vi "find_rects_test.vi"() -> ()   [LabVIEW 2023]
uses:
  find_rects_parameters.ctl
  Vision.lvlib
panel:
  out "rects":T1(array[cluster]) {"x" format="%#_3g"; "y" format="%#_3g"; "width" format="%#_3g"; "height" format="%#_3g"; "angle" format="%#_3g"; "image-x" format="%#_3g"; "image-y" format="%#_3g"}
  in  "find_rects parameters":T2={"nominalWidth"=1.0, "nominalHeight"=1.0, "tolerance"=0.5, "pointSelect"=4.0, "allowRotation"=FALSE}
  in  "Field of View":cluster{"fieldOfViewX":sgl, "fieldOfViewY":sgl}={"fieldOfViewX"=1.4, "fieldOfViewY"=1.048}
  out "Number of Rects":i32
  in  "File Path":path=path "C:/Users/Caleb/Downloads/fid_range_test_br_7.png"
  out "error out":errorcluster
  out "Image":T3(plugin-control)
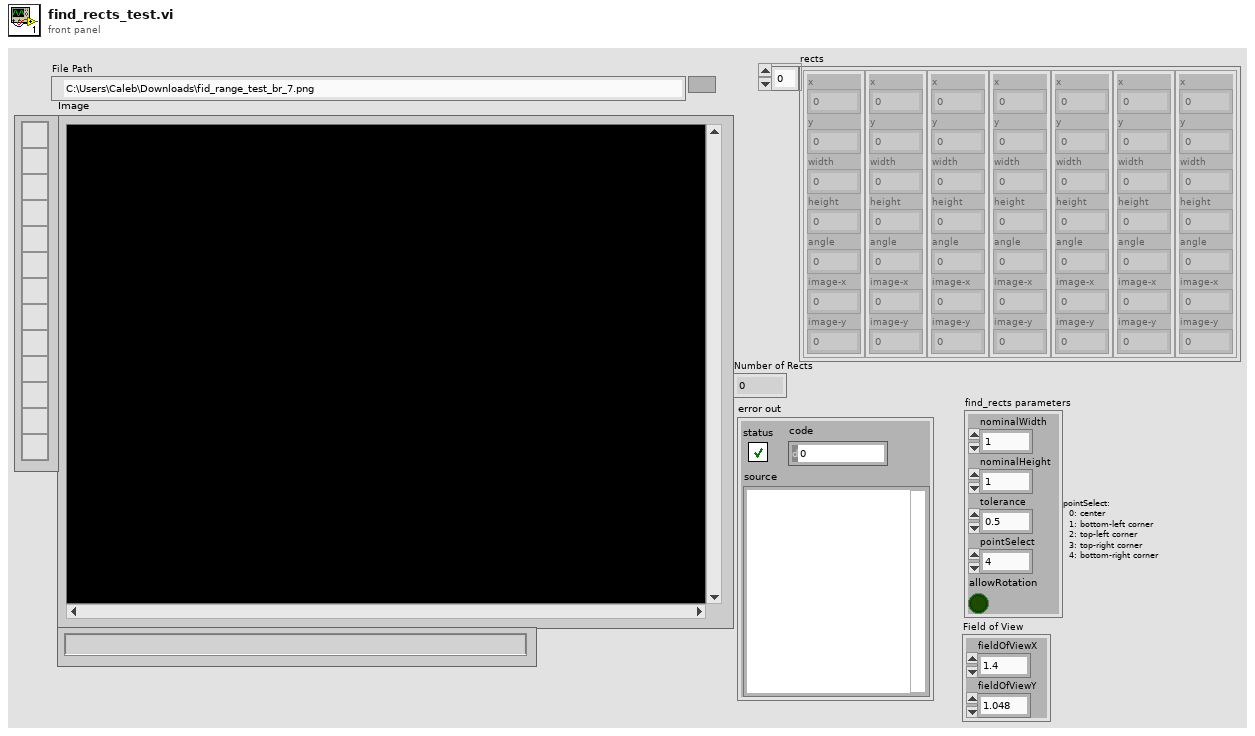
[diagram p1: front panel]
types:
  T1 = cluster{"x":dbl, "y":dbl, "width":dbl, "height":dbl, "angle":dbl, "image-x":dbl, "image-y":dbl}[]
  T2 = typedef "Vision.lvlib/find_rects_parameters.ctl" = cluster{"nominalWidth":sgl, "nominalHeight":sgl, "tolerance":sgl, "pointSelect":sgl, "allowRotation":bool}
  T3 = typedef "IMAQ Image.ctl" = refnum<image>
  T4 = cluster{"Left":i32, "Top":i32, "Right":i32, "Bottom":i32}
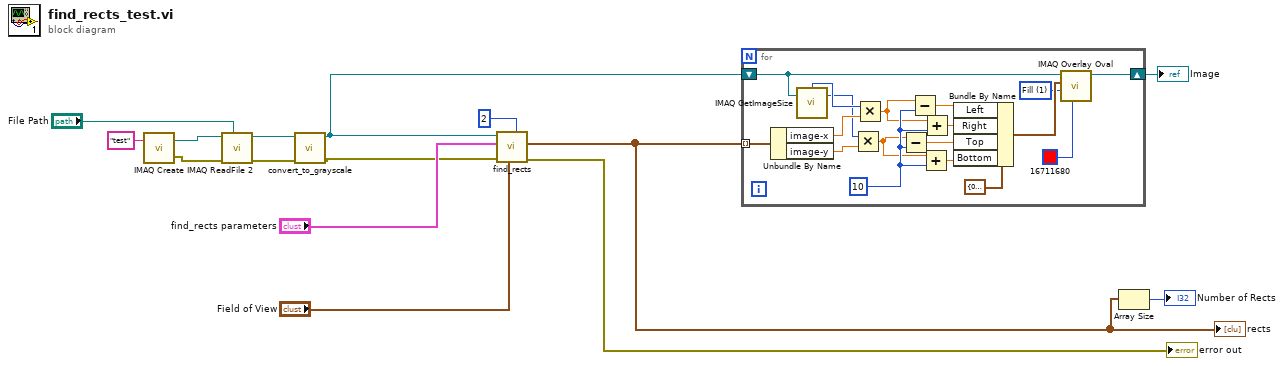
[diagram p0: block diagram]
diagram:
  n1 = call "IMAQ Create"("Image Name"="test") -> ("New Image"=w15:T3, "error out"=w13:errorcluster)  [unwired: 4 in]
  n2 = call "IMAQ ReadFile 2"("File Path"="File Path", "error in (no error)"=w13, "Image"=w15) -> ("error out"=w1:errorcluster, "Image Out"=w4:T3)  [unwired: 4 in, 3 out]
  n3 = call "convert_to_grayscale.vi"("error in (no error)"=w1, "Image in"=w4) -> ("error out"=w2:errorcluster, "Image out"=w3:T3)  [unwired: 8 in]
  n4 = call "find_rects.vi"("shrinkFactor"=2 ("Shrink Factor"), "Field of View"="Field of View", "error in"=w2, "find_patches parameters"="find_rects parameters", "Image"=w3) -> ("error out"=→"error out":errorcluster, "rects"=w5:T1)  [unwired: 5 in]
  "rects" <- w5
  n5 = for {
    shift-right: [w18] -> w7
    shift-left: w3 -> [w29]
    tunnel: w5 -> [w16] mode=indexing
    w17 = u32 1 items=["Frame", "Fill"] ("Drawing Mode (Frame)")
    w22 = 10
    n6 = Unbundle By Name(w16) -> ("image-x"=w33:dbl, "image-y"=w31:dbl)
    n7 = call "IMAQ GetImageSize"("Image"=w29) -> ("Y Resolution"=w30:i32, "X Resolution"=w32:i32)  [unwired: 3 in, 1 out]
    n8 = Multiply(x=w30, y=w31) -> (x*y=w21:dbl)
    n9 = Multiply(x=w32, y=w33) -> (x*y=w20:dbl)
    n10 = Subtract(x=w21, y=w22) -> (x-y=w23:dbl)
    n11 = Subtract(x=w20, y=w22) -> (x-y=w24:dbl)
    n12 = Add(x=w21, y=w22) -> (x+y=w25:dbl)
    n13 = Add(x=w20, y=w22) -> (x+y=w26:dbl)
    n14 = Bundle By Name(cluster=T4 {"Left"=0, "Top"=0, "Right"=0, "Bottom"=0} ("Bounding Rectangle"), "Left"=w24, "Right"=w26, "Top"=w23, "Bottom"=w25) -> (w19:T4)
    n15 = call "IMAQ Overlay Oval"("Color"=u32 16711680, "Drawing Mode (Frame)"=w17, "Bounding Rectangle"=w19, "Image"=w29) -> ("Image Out"=w18:T3)  [unwired: 6 in, 1 out]
  }
  "Image" <- w7
  n16 = Array Size(array=w5) -> (size(s)=→"Number of Rects":i32)
